vi "Read PCBAID.vi"(11 "Error In":errorcluster) -> (4 "PCBA ID":i32, 8 "Console text":string, 15 "Error Out":errorcluster)   [LabVIEW 2021]
doc: "Gets the PCBA ID by calling a Python script which uses PCAN USB1 to read it from this frame: \n\nBO_ 2420637697 IPC_AppData_0: 8 IPC\n SG_ IPC_MetaVersion : 0|16@1+ (1,0) [0|65535] \"\" HC\n SG_ IPC_MCU_ID : 16|16@1+ (1,0) [0|65535] \"\" HC\n SG_ IPC_PCBA_ID : 32|16@1+ (1,0) [0|65535] \"\" HC\n SG_ IPC_Config_ID : 48|16@1+ (1,0) [0|65535] \"\" HC"
uses:
  <vilib>/regexp/Match Regular Expression.xnode
panel:
  # "Inputs"
  # "Outputs"
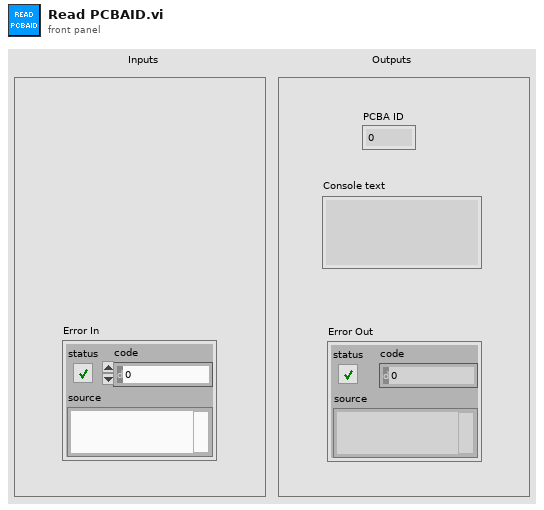
[diagram p1: front panel]
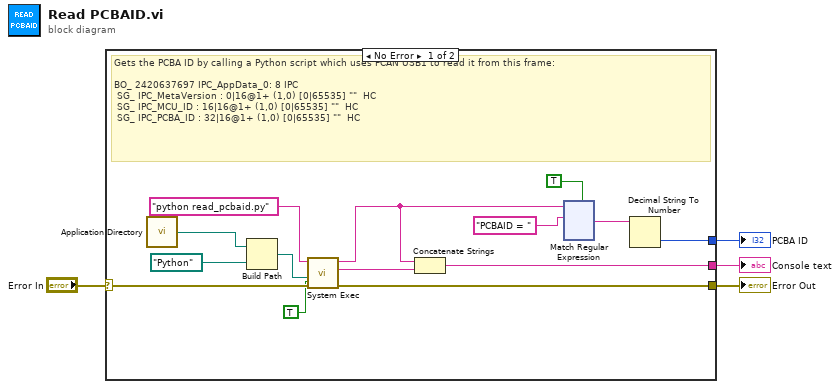
[diagram p0: block diagram]
diagram:
  n1 = case shown="No Error" "Error In" {
    selector: "Error In" -> [w17 w136]
    tunnel: [w10 w136] -> w3
    tunnel: [w7 _] -> w2
    tunnel: [w6 _] -> w1
    frame No Error {
      # "Gets the PCBA ID by calling a Python script which uses PCAN USB1 to read it from this frame: \n\nBO_ 2420637697 IPC_AppData_0: 8 IPC\n SG_ IPC_MetaVersion : 0|16@1+ (1,0) [0|65535] \"\"  HC\n SG_ IPC_MCU_ID : 16|16@1+ (1,0) [0|65535] \"\"  HC\n SG_ IPC_PCBA_ID : 32|16@1+ (1,0) [0|65535] \"\"  HC"
      n2 = call <vilib>:"Application Directory.vi"() -> ("Application Directory"=w16:path)
      n3 = Build Path(base path=w16, name or relative path=path "Python") -> (appended path=w14:path)
      n4 = call <vilib>:"System Exec.vi"("run minimized? (F)"=TRUE, "error in (no error)"=w17, "working directory"=w14, "command line"="python read_pcbaid.py") -> ("error out"=w10:errorcluster, "standard error"=w5:string, "standard output"=w9:string)  [unwired: 4 in, 1 out]
      n5 = Concatenate Strings(w9, w5) -> (w6:string)
      n6 = xnode "Match Regular Expression"("input string"=w9, "regular expression"="PCBAID = " ("search string/char (-)"), "multiline? (F)"=TRUE) -> ("after match"=w8:string)  [unwired: 3 in, 4 out]
      n7 = Decimal String To Number(string=w8) -> (number=w7:i32)  [unwired: 2 in, 1 out]
    }
    frame Error {
      # "Can't start due to error"
    }
  }
  "Error Out" <- w3
  "PCBA ID" <- w2
  "Console text" <- w1
